vi "Stoermeldung blinken lassen.vi"(8 "error in (no error)":errorcluster caption="Fehler (Eingang, kein Fehler)", 11 "Fehler steht an":bool) -> (0 "error out":errorcluster caption="Fehler (Ausgang)", 3 "Blinken":bool)   [LabVIEW 2020, in "Allgemein.lvlib"]
uses:
  Allgemein.lvlib
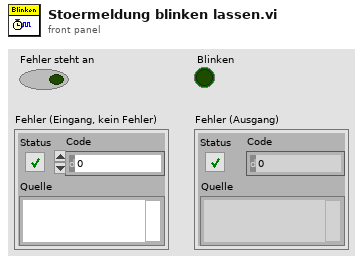
[diagram p1: front panel]
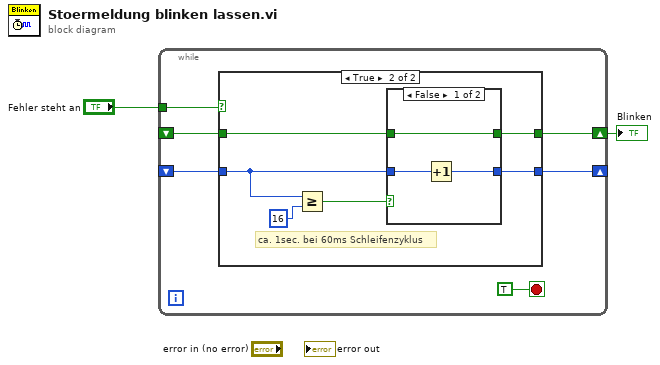
[diagram p0: block diagram]
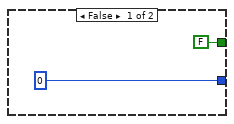
[diagram p2: hidden frame]
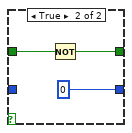
[diagram p3: hidden frame]
diagram:
  n1 = while {
    shift-right: [w7] -> _
    shift-left: _ -> [w6]
    tunnel: "Fehler steht an" -> [w4]
    shift-right: [w5] -> w1
    shift-left: _ -> [w3]
    stop <- TRUE stop-if-true
    n2 = case shown="True" w4 {
      tunnel: [0 w16] -> w7
      tunnel: w6 -> [_ w13]
      tunnel: [FALSE w12] -> w5
      tunnel: w3 -> [_ w11]
      frame False {
      }
      frame True {
        # "ca. 1sec. bei 60ms Schleifenzyklus"
        n3 = Greater Or Equal?(x=w13, y=16) -> (x >= y?=w14:bool)
        n4 = case shown="False" w14 {
          tunnel: [w18 0] -> w16
          tunnel: w13 -> [w19 _]
          tunnel: [w17 w21] -> w12
          tunnel: w11 -> [w17 w20]
          frame False {
            n5 = Increment(x=w19) -> (x+1=w18:i32)
          }
          frame True {
            n6 = Not(x=w20) -> (.not. x?=w21:bool)
          }
        }
      }
    }
  }
  "Blinken" <- w1
